vi "Select First Tree Item.vi"(8 "error in (no error)":errorcluster, 11 "TreeControl in":refnum<vi>) -> (0 "error out":errorcluster, 3 "reference out":refnum<vi>)   [LabVIEW 2021, in "Seq Edit Quick Drop.lvlib"]
uses:
  Seq Edit Quick Drop.lvlib
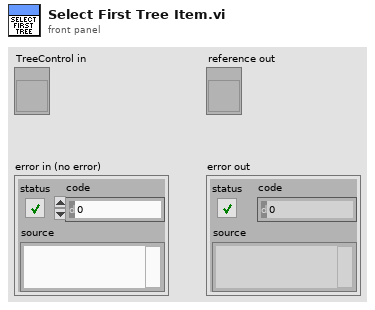
[diagram p1: front panel]
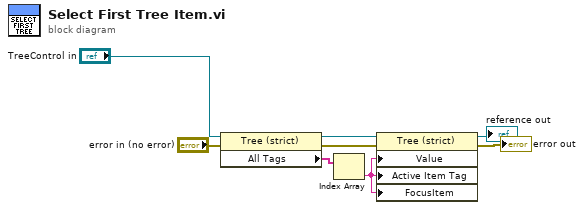
[diagram p0: block diagram]
diagram:
  n1 = property class="Tree (strict)"(reference="TreeControl in", error in="error in (no error)") -> (reference out=w2:refnum<vi>, error out=w3:errorcluster, "All Tags"=w7:string[])
  n2 = Index Array(array=w7) -> (element=w5:string)  [unwired: 1 in]
  n3 = property class="Tree (strict)"(reference=w2, error in=w3, "Value"=w5, "Active Item Tag"=w5, "FocusItem"=w5) -> (reference out=→"reference out":refnum<vi>, error out=→"error out":errorcluster)
